vi "Smooth_Image_Edge_Detect.vi"(3 "Edge detection weight parameter":dbl=0.1, 4 "Preserve size? (F)":bool, 5 "Edge output? (F)":bool, 6 "Input Image Pixels (U32)":u32[][](array[numeric])) -> (1 "Output image size":i32[](array[numeric]), 2 "Output Image Pixels (U32)":u32[][](array[numeric]))   [LabVIEW 2018]
uses:
  <vilib>/Analysis/2dsp.llb/2D Convolution (DBL).vi
  <vilib>/Analysis/NI_AALPro.lvlib
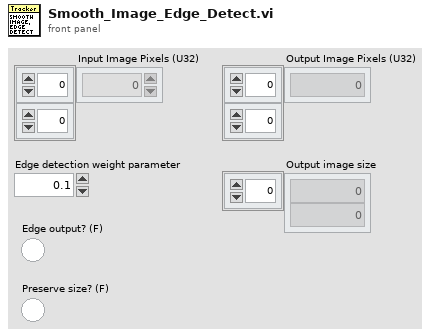
[diagram p1: front panel]
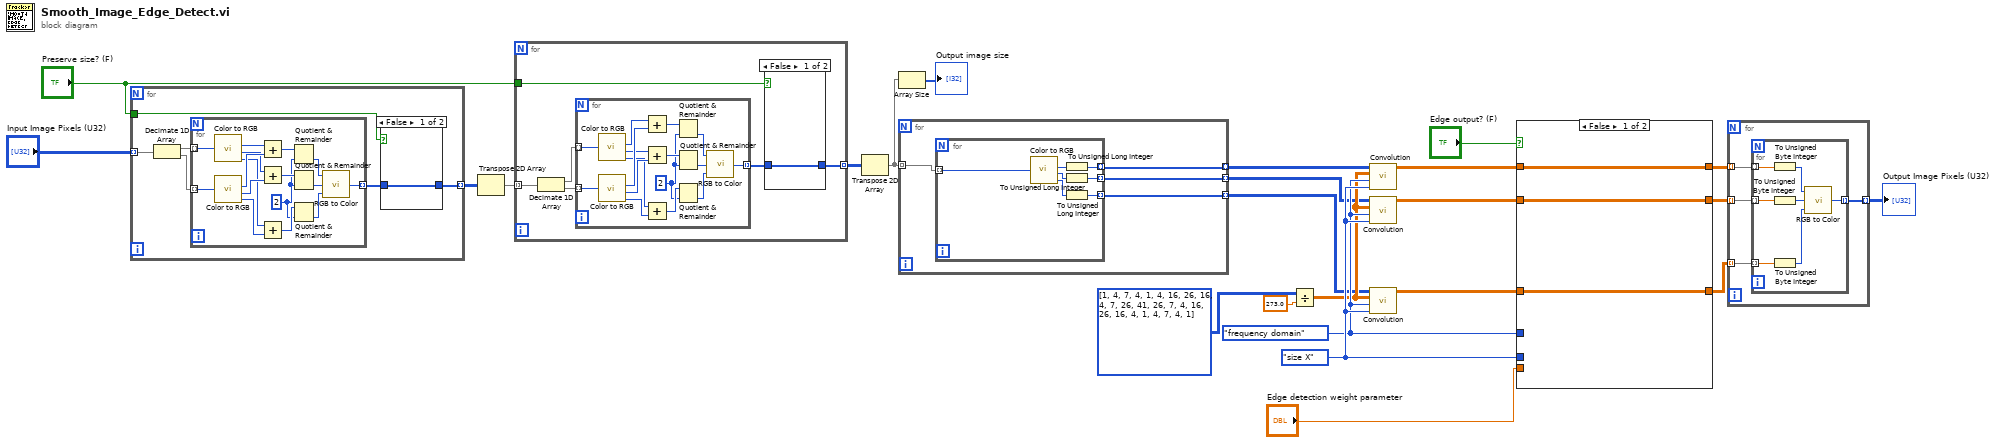
[diagram p0: block diagram]
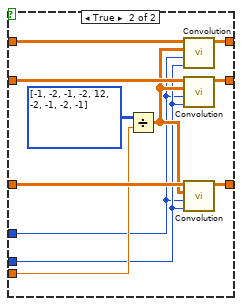
[diagram p2: hidden frame]
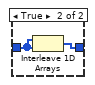
[diagram p3: hidden frame]
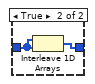
[diagram p4: hidden frame]
diagram:
  w16 = enum32{"direct", "frequency domain"}."frequency domain" ("algorithm")
  w17 = enum32{"full", "size X", "compact"}."size X" ("output size")
  n1 = for {
    tunnel: "Input Image Pixels (U32)" -> [w30] mode=indexing
    tunnel: [w26] -> w4 mode=indexing
    tunnel: "Preserve size? (F)" -> [w25]
    n2 = Decimate 1D Array(w30) -> (w28:u32[], w29:u32[])
    n3 = for {
      tunnel: w29 -> [w48] mode=indexing
      tunnel: w28 -> [w49] mode=indexing
      tunnel: [w34] -> w27 mode=indexing
      w44 = u32 2
      n4 = call <vilib>:"Color to RGB.vi"("Color"=w49) -> ("R"=w43:u8, "G"=w41:u8, "B"=w39:u8)  [unwired: 1 out]
      n5 = call <vilib>:"Color to RGB.vi"("Color"=w48) -> ("R"=w42:u8, "G"=w40:u8, "B"=w38:u8)  [unwired: 1 out]
      n6 = Add(x=w43, y=w42) -> (x+y=w47:u32)
      n7 = Add(x=w41, y=w40) -> (x+y=w46:u32)
      n8 = Add(x=w39, y=w38) -> (x+y=w45:u32)
      n9 = Quotient & Remainder(x=w47, y=w44) -> (floor(x/y)=w37:u32)  [unwired: 1 out]
      n10 = Quotient & Remainder(x=w46, y=w44) -> (floor(x/y)=w36:u32)  [unwired: 1 out]
      n11 = Quotient & Remainder(x=w45, y=w44) -> (floor(x/y)=w35:u32)  [unwired: 1 out]
      n12 = call <vilib>:"RGB to Color.vi"("B"=w35, "G"=w36, "R"=w37) -> ("Color"=w34:u32)
    }
    n13 = case shown="False" w25 {
      tunnel: w27 -> [w31 w33]
      tunnel: [w31 w32] -> w26
      frame False {
      }
      frame True {
        n14 = Interleave 1D Arrays(w33, w33) -> (w32:u32[])
      }
    }
  }
  n15 = Transpose 2D Array(2D array=w4) -> (transposed array=w5:u32[][])
  n16 = for {
    tunnel: w5 -> [w55] mode=indexing
    tunnel: [w51] -> w6 mode=indexing
    tunnel: "Preserve size? (F)" -> [w50]
    n17 = Decimate 1D Array(w55) -> (w53:u32[], w54:u32[])
    n18 = for {
      tunnel: w54 -> [w73] mode=indexing
      tunnel: w53 -> [w74] mode=indexing
      tunnel: [w59] -> w52 mode=indexing
      w69 = u32 2
      n19 = call <vilib>:"Color to RGB.vi"("Color"=w74) -> ("R"=w68:u8, "G"=w66:u8, "B"=w64:u8)  [unwired: 1 out]
      n20 = call <vilib>:"Color to RGB.vi"("Color"=w73) -> ("R"=w67:u8, "G"=w65:u8, "B"=w63:u8)  [unwired: 1 out]
      n21 = Add(x=w68, y=w67) -> (x+y=w72:u32)
      n22 = Add(x=w66, y=w65) -> (x+y=w71:u32)
      n23 = Add(x=w64, y=w63) -> (x+y=w70:u32)
      n24 = Quotient & Remainder(x=w72, y=w69) -> (floor(x/y)=w62:u32)  [unwired: 1 out]
      n25 = Quotient & Remainder(x=w71, y=w69) -> (floor(x/y)=w61:u32)  [unwired: 1 out]
      n26 = Quotient & Remainder(x=w70, y=w69) -> (floor(x/y)=w60:u32)  [unwired: 1 out]
      n27 = call <vilib>:"RGB to Color.vi"("B"=w60, "G"=w61, "R"=w62) -> ("Color"=w59:u32)
    }
    n28 = case shown="False" w50 {
      tunnel: w52 -> [w56 w58]
      tunnel: [w56 w57] -> w51
      frame False {
      }
      frame True {
        n29 = Interleave 1D Arrays(w58, w58) -> (w57:u32[])
      }
    }
  }
  n30 = Transpose 2D Array(2D array=w6) -> (transposed array=w13:u32[][])
  n31 = Array Size(array=w13) -> (size(s)=→"Output image size":i32[])
  n32 = for {
    tunnel: w13 -> [w78] mode=indexing
    tunnel: [w77] -> w8 mode=indexing
    tunnel: [w76] -> w9 mode=indexing
    tunnel: [w75] -> w10 mode=indexing
    n33 = for {
      tunnel: w78 -> [w85] mode=indexing
      tunnel: [w81] -> w77 mode=indexing
      tunnel: [w80] -> w76 mode=indexing
      tunnel: [w79] -> w75 mode=indexing
      n34 = call <vilib>:"Color to RGB.vi"("Color"=w85) -> ("R"=w84:u8, "G"=w83:u8, "B"=w82:u8)  [unwired: 1 out]
      n35 = To Unsigned Long Integer(number=w84) -> (unsigned 32bit integer=w81:u32)
      n36 = To Unsigned Long Integer(number=w83) -> (unsigned 32bit integer=w80:u32)
      n37 = To Unsigned Long Integer(number=w82) -> (unsigned 32bit integer=w79:u32)
    }
  }
  n38 = Divide(x=i32[][] [[1, 4, 7, 4, 1], [4, 16, 26, 16, 4], [7, 26, 41, 26, 7], [4, 16, 26, 16, 4], [1, 4, 7, 4, 1]], y=273.0) -> (x/y=w11:dbl[][])
  n39 = call-poly <vilib>:"Convolution.vi"("output size"=w17, "algorithm"=w16, "Y"=w11, "X"=w8) -> ("X * Y"=w19:dbl[][])  [unwired: 6 in, 1 out]
  n40 = call-poly <vilib>:"Convolution.vi"("output size"=w17, "algorithm"=w16, "Y"=w11, "X"=w9) -> ("X * Y"=w20:dbl[][])  [unwired: 6 in, 1 out]
  n41 = call-poly <vilib>:"Convolution.vi"("output size"=w17, "algorithm"=w16, "Y"=w11, "X"=w10) -> ("X * Y"=w21:dbl[][])  [unwired: 6 in, 1 out]
  n42 = case shown="False" "Edge output? (F)" {
    tunnel: [w86 w99] -> w24
    tunnel: [w87 w98] -> w23
    tunnel: [w88 w97] -> w22
    tunnel: w21 -> [w86 w96]
    tunnel: w20 -> [w87 w95]
    tunnel: w19 -> [w88 w94]
    tunnel: "Edge detection weight parameter" -> [_ w92]
    tunnel: w17 -> [_ w90]
    tunnel: w16 -> [_ w89]
    frame False {
    }
    frame True {
      n43 = Divide(x=i32[][] [[-1, -2, -1], [-2, 12, -2], [-1, -2, -1]], y=w92) -> (x/y=w93:dbl[][])
      n44 = call-poly <vilib>:"Convolution.vi"("output size"=w90, "algorithm"=w89, "Y"=w93, "X"=w94) -> ("X * Y"=w97:dbl[][])  [unwired: 6 in, 1 out]
      n45 = call-poly <vilib>:"Convolution.vi"("output size"=w90, "algorithm"=w89, "Y"=w93, "X"=w95) -> ("X * Y"=w98:dbl[][])  [unwired: 6 in, 1 out]
      n46 = call-poly <vilib>:"Convolution.vi"("output size"=w90, "algorithm"=w89, "Y"=w93, "X"=w96) -> ("X * Y"=w99:dbl[][])  [unwired: 6 in, 1 out]
    }
  }
  n47 = for {
    tunnel: w22 -> [w103] mode=indexing
    tunnel: w23 -> [w102] mode=indexing
    tunnel: w24 -> [w101] mode=indexing
    tunnel: [w100] -> w12 mode=indexing
    n48 = for {
      tunnel: w103 -> [w110] mode=indexing
      tunnel: w102 -> [w109] mode=indexing
      tunnel: w101 -> [w108] mode=indexing
      tunnel: [w104] -> w100 mode=indexing
      n49 = To Unsigned Byte Integer(number=w110) -> (unsigned 8bit integer=w107:u8)
      n50 = To Unsigned Byte Integer(number=w109) -> (unsigned 8bit integer=w106:u8)
      n51 = To Unsigned Byte Integer(number=w108) -> (unsigned 8bit integer=w105:u8)
      n52 = call <vilib>:"RGB to Color.vi"("B"=w105, "G"=w106, "R"=w107) -> ("Color"=w104:u32)
    }
  }
  "Output Image Pixels (U32)" <- w12
